vi "Init.vi"(0 "InfluxDB in":refnum<class "InfluxDB Client.lvclass">, 5 "Url":string, 7 "Username":string, 9 "Password":string, 11 "error in (no error)":errorcluster) -> (4 "InfluxDB out":refnum<class "InfluxDB Client.lvclass">, 15 "error out":errorcluster)   [LabVIEW 2013, in "InfluxDB Client.lvclass"]
doc: "Initializes the InfluxDB client."
uses:
  InfluxDB Client.lvclass
  InfluxDB Client.lvclass/InfluxDB Client.ctl
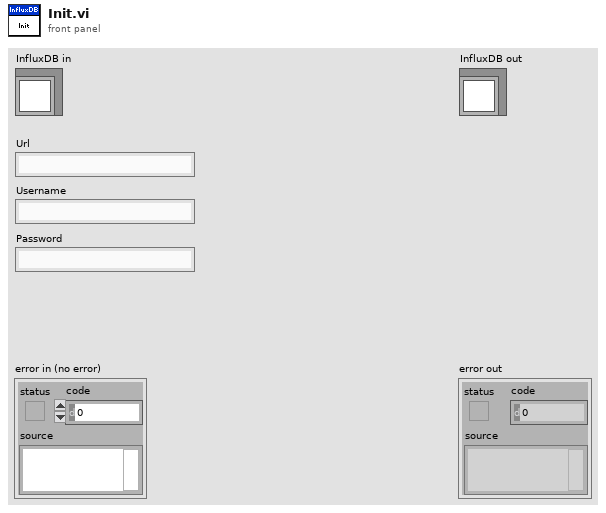
[diagram p1: front panel]
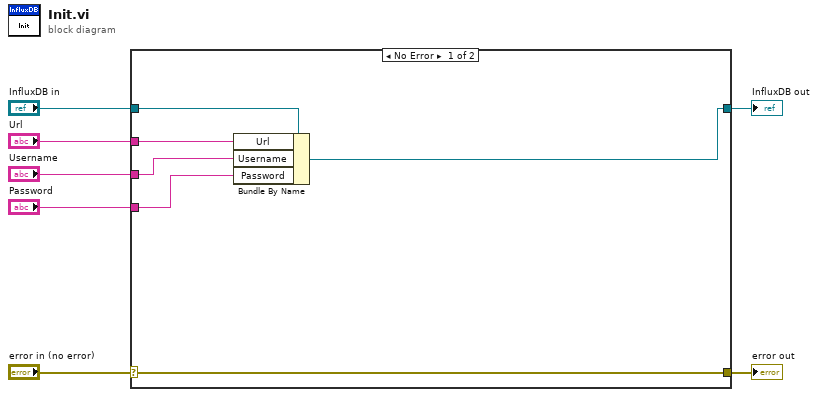
[diagram p0: block diagram]
diagram:
  n1 = case shown="No Error" "error in (no error)" {
    selector: "error in (no error)" -> [w13 w15]
    tunnel: [w13 w15] -> w6
    tunnel: [w11 w14] -> w4
    tunnel: "InfluxDB in" -> [w12 w14]
    tunnel: "Url" -> [w10 _]
    tunnel: "Username" -> [w9 _]
    tunnel: "Password" -> [w8 _]
    frame No Error {
      n2 = Bundle By Name(cluster=w12, "Url"=w10, "Username"=w9, "Password"=w8) -> (w11:refnum<class "InfluxDB Client.lvclass">)
    }
    frame Error {
    }
  }
  "error out" <- w6
  "InfluxDB out" <- w4
